vi "Inv Normal Distribution.vi"(0 "probability":dbl format="%0.4f") -> (1 "x":dbl format="%0.4f", 2 "error":i32)   [LabVIEW 2017, in "NI_AALPro.lvlib"]
doc: "LabVIEW no longer supports this VI. Use the Continuous Inverse CDF VI (Normal instance) instead. Computes the value of <B>x</B> given the <B>probability</B> value, p, of a Normally distributed random variable, X. The Inv Normal Distribution VI computes the value of <B>x</B> such that the following condition is satisfied: p = Prob{X <= <B>x</B>}, where X is standard Normally distributed, p is the <B>probability</B>, and <B>x</B> is the value."
uses:
  NI_AALPro.lvlib
  <resource>/lvanlys.dll
panel:
  # "Inverse Normal\n  Distribution"
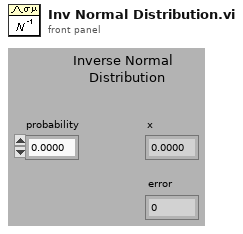
[diagram p1: front panel]
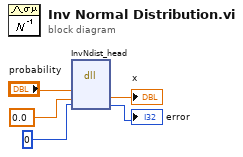
[diagram p0: block diagram]
diagram:
  n1 = dll-call lib="C:/Program Files (x86)/National Instruments/LabVIEW 2017/resource/lvanlys.*" fn="InvNdist_head"("probability"="probability", 0.0, 0) -> (→"x":dbl, →"error":i32)  [unwired: 5 in, 2 out]
